vi "Get Value.vi"(11 "CANopen Message":refnum<class "CANopen Message.lvclass">) -> (3 "Value":u8[](array[numeric]))   [LabVIEW 2024, in "CANopen Master.lvlib" / "Service Data Object.lvclass"]
uses:
  Service Data Object.lvclass
  Service Data Object.lvclass/Service Data Object.ctl
  CANopen Message/CANopen Message.lvclass
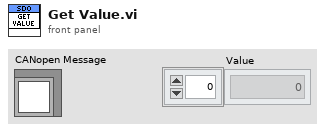
[diagram p1: front panel]
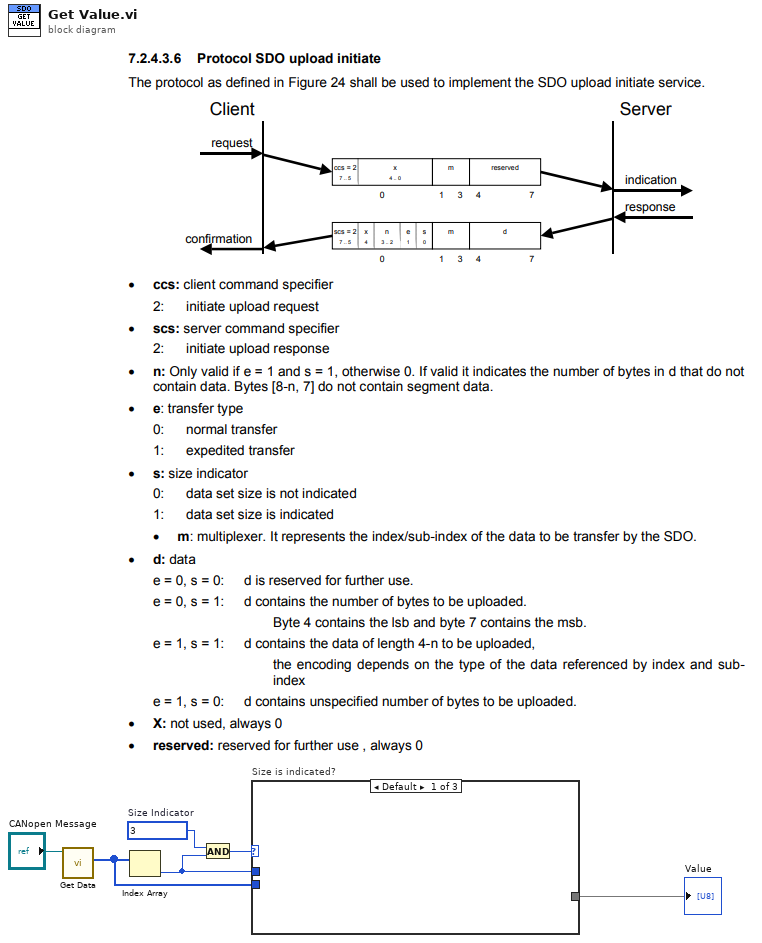
[diagram p0: block diagram]
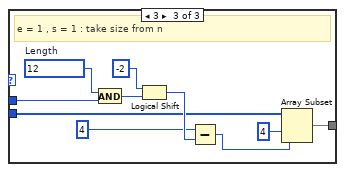
[diagram p3: hidden frame]
diagram:
  w5 = u8 3  # Size Indicator
  n1 = call "Get Data.vi"("CANopen Message in"="CANopen Message") -> ("Data"=w2:u8[])  [unwired: 9 in, 1 out]
  n2 = Index Array(array=w2) -> (element=w3:u8)  [unwired: 1 in]
  n3 = And(x=w5, y=w3) -> (x .and. y?=w4:u8)
  n4 = case "Size is indicated?" shown="Default" w4 {
    tunnel: w3 -> [_ _ w16]
    tunnel: w2 -> [_ _ w11]
    tunnel: [_ _ w8] -> w1
    frame Default {
    }
    frame 1 {
      # "e = 0, s = 1\nd contains the number of byte to be uploaded"
    }
    frame 3 {
      w15 = u8 12  # Length
      # "e = 1 , s = 1 : take size from n"
      n5 = And(x=w15, y=w16) -> (x .and. y?=w14:u8)
      n6 = Logical Shift(y=i16 -2, x=w14) -> (x << y=w12:u8)
      n7 = Subtract(x=4 ("index"), y=w12) -> (x-y=w9:i32)
      n8 = Array Subset(array=w11, index=4, length=w9) -> (w8:u8[])
    }
  }
  "Value" <- w1
